vi "Build Order.vi"(8 "error in (no error)":errorcluster, 9 "Customer Name":string, 10 "Customer":refnum<class "Customer.lvclass">, 11 "Order":cluster{"Drink type":T1, "Options":T2[]}[](array[cluster])) -> (0 "error out":errorcluster, 3 "Order Out":refnum<class "Order.lvclass">)   [LabVIEW 2020, in "Order.lvclass"]
doc: "Generate and initialize an Order object."
uses:
  Order.lvclass
  Beverages/TypeDefs/Drink Type.ctl
  Beverages/TypeDefs/Options.ctl
  Processes/People/Customers/Customer/Customer.lvclass
  Beverages/Beverage/Beverage.lvclass
  Beverages/Beverage/Beverage.lvclass/Beverage.ctl
  Order.lvclass/Order.ctl
  Beverages/Beverage/Write Drink Type.vi
  Beverages/Beverage/Write Options.vi
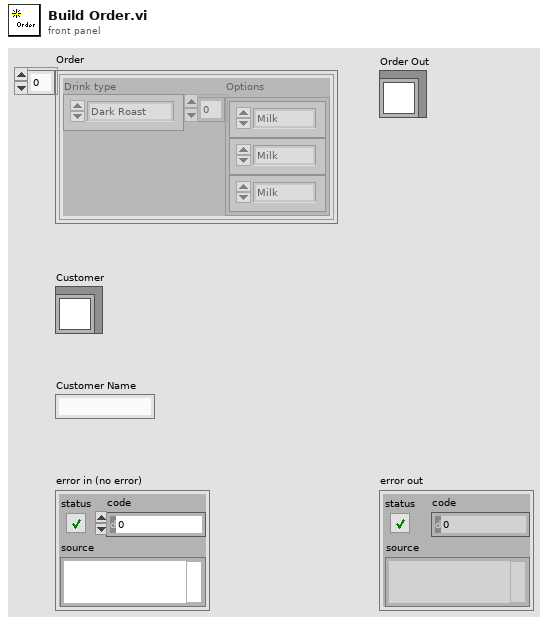
[diagram p1: front panel]
types:
  T1 = typedef "Beverage.lvclass/Drink Type.ctl" = enum16{"Dark Roast", "Decaf", "Espresso", "House Blend"}
  T2 = typedef "Beverage.lvclass/Options.ctl" = enum16{"<None>", "Milk", "Mocha", "Soy", "Whip"}
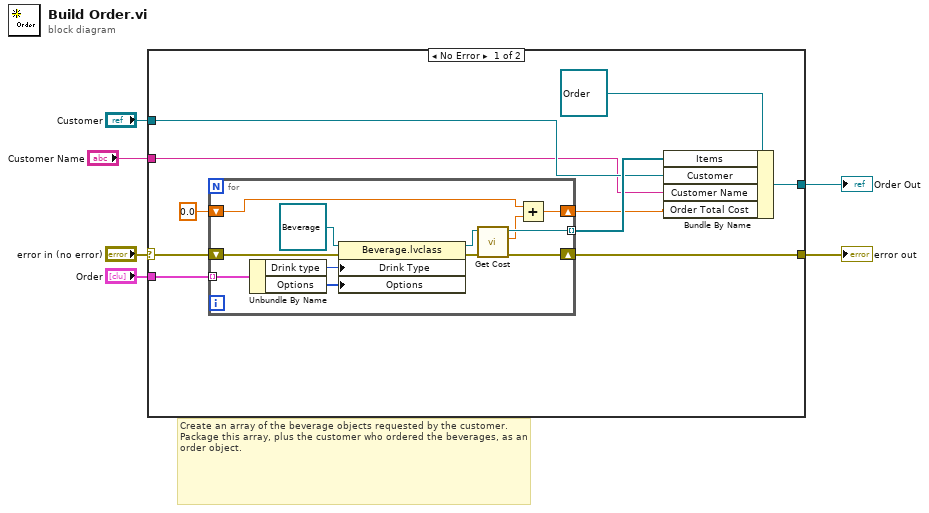
[diagram p0: block diagram]
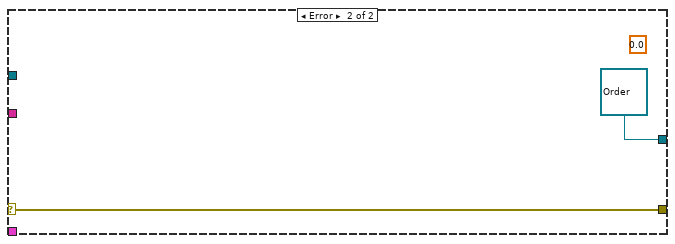
[diagram p2: hidden frame]
diagram:
  # "Create an array of the beverage objects requested by the customer.  Package this array, plus the customer who ordered the beverages, as an order object."
  n1 = case shown="No Error" "error in (no error)" {
    selector: "error in (no error)" -> [w10 w30]
    tunnel: "Order" -> [w16 _]
    tunnel: [w13 refnum<class "Order.lvclass"> refnum ("Order.lvclass")] -> w5
    tunnel: "Customer" -> [w12 _]
    tunnel: [w9 w30] -> w2
    tunnel: "Customer Name" -> [w8 _]
    frame No Error {
      n2 = for {
        tunnel: w16 -> [w28] mode=indexing
        tunnel: [w27] -> w14 mode=indexing
        shift-right: [w26] -> w7
        shift-left: 0.0 -> [w24]
        shift-right: [w17] -> w9
        shift-left: w10 -> [w18]
        n3 = Unbundle By Name(w28) -> ("Drink type"=w22:T1, "Options"=w21:T2[])
        n4 = property on="Property Node" class="Beverage.lvclass"(reference=refnum<class "Beverage.lvclass"> refnum ("Beverage in"), error in=w18, "Drink Type"=w22, "Options"=w21) -> (reference out=w20:refnum<class "Beverage.lvclass">, error out=w19:errorcluster)
        n5 = call "Get Cost.vi"("error in (no error)"=w19, "Beverage in"=w20) -> ("error out"=w17:errorcluster, "Cost"=w25:dbl, "Beverage out"=w27:refnum<class "Beverage.lvclass">)  [unwired: 7 in]
        n6 = Add(x=w24, y=w25) -> (x+y=w26:dbl)
      }
      n7 = Bundle By Name(cluster=refnum<class "Order.lvclass"> refnum ("Order.lvclass"), "Items"=w14, "Customer"=w12, "Customer Name"=w8, "Order Total Cost"=w7) -> (w13:refnum<class "Order.lvclass">)
    }
    frame Error {
      (unwired) 0.0
    }
  }
  "Order Out" <- w5
  "error out" <- w2
